vi "extract central core for intensity.vi"() -> ()   [LabVIEW 2020]
uses:
  <vilib>/Math Plots/3D Math Plots/3D Surface/3D Surface XCtrl/3D Surface.xctl
  <vilib>/Math Plots/3D Math Plots/3D Surface/3D Surface Datatype/Public/Plot Helper (Vector).vi
  <vilib>/Math Plots/3D Math Plots/3D Surface/3D Surface Datatype/3D Surface Datatype.lvclass
panel:
  in  "Offset Dim 2":i32
  in  "Offset Dim 1":i32
  out "Main Image 2":T1(plugin-control)
  out "Core Image":T1(plugin-control)
  in  "Boolean":bool
  out "3D Surface":refnum<class "3D Plot Datatype.lvclass">[](xcontrol)
  in  "Intensity Graph colour palette":cluster{dbl, "Color Box":u32}[](array[cluster])=[{1000.0, "Color Box"=16714752}, {750.0, "Color Box"=15859456}, {500.0, "Color Box"=65289}, {250.0, "Color Box"=983260}, {0.0, "Color Box"=14418124}]
  out "output array":i16[](array[numeric])
  out "Intensity Graph 3":i16[][](graph)
  out "dim2_length":i32
  out "dim2_start":i32
  out "dim1_length":i32
  out "dim1_start":i32
  in  "Core extraction size":i32
  out "output variable 6":dbl
  out "output variable 5":dbl
  out "output variable 4":dbl
  out "output variable 3":dbl
  out "output variable 2":i32
  out "output variable":i32
  out "size(s)":i32[](array[numeric])
  out "Intensity Graph 2":i16[][](graph)
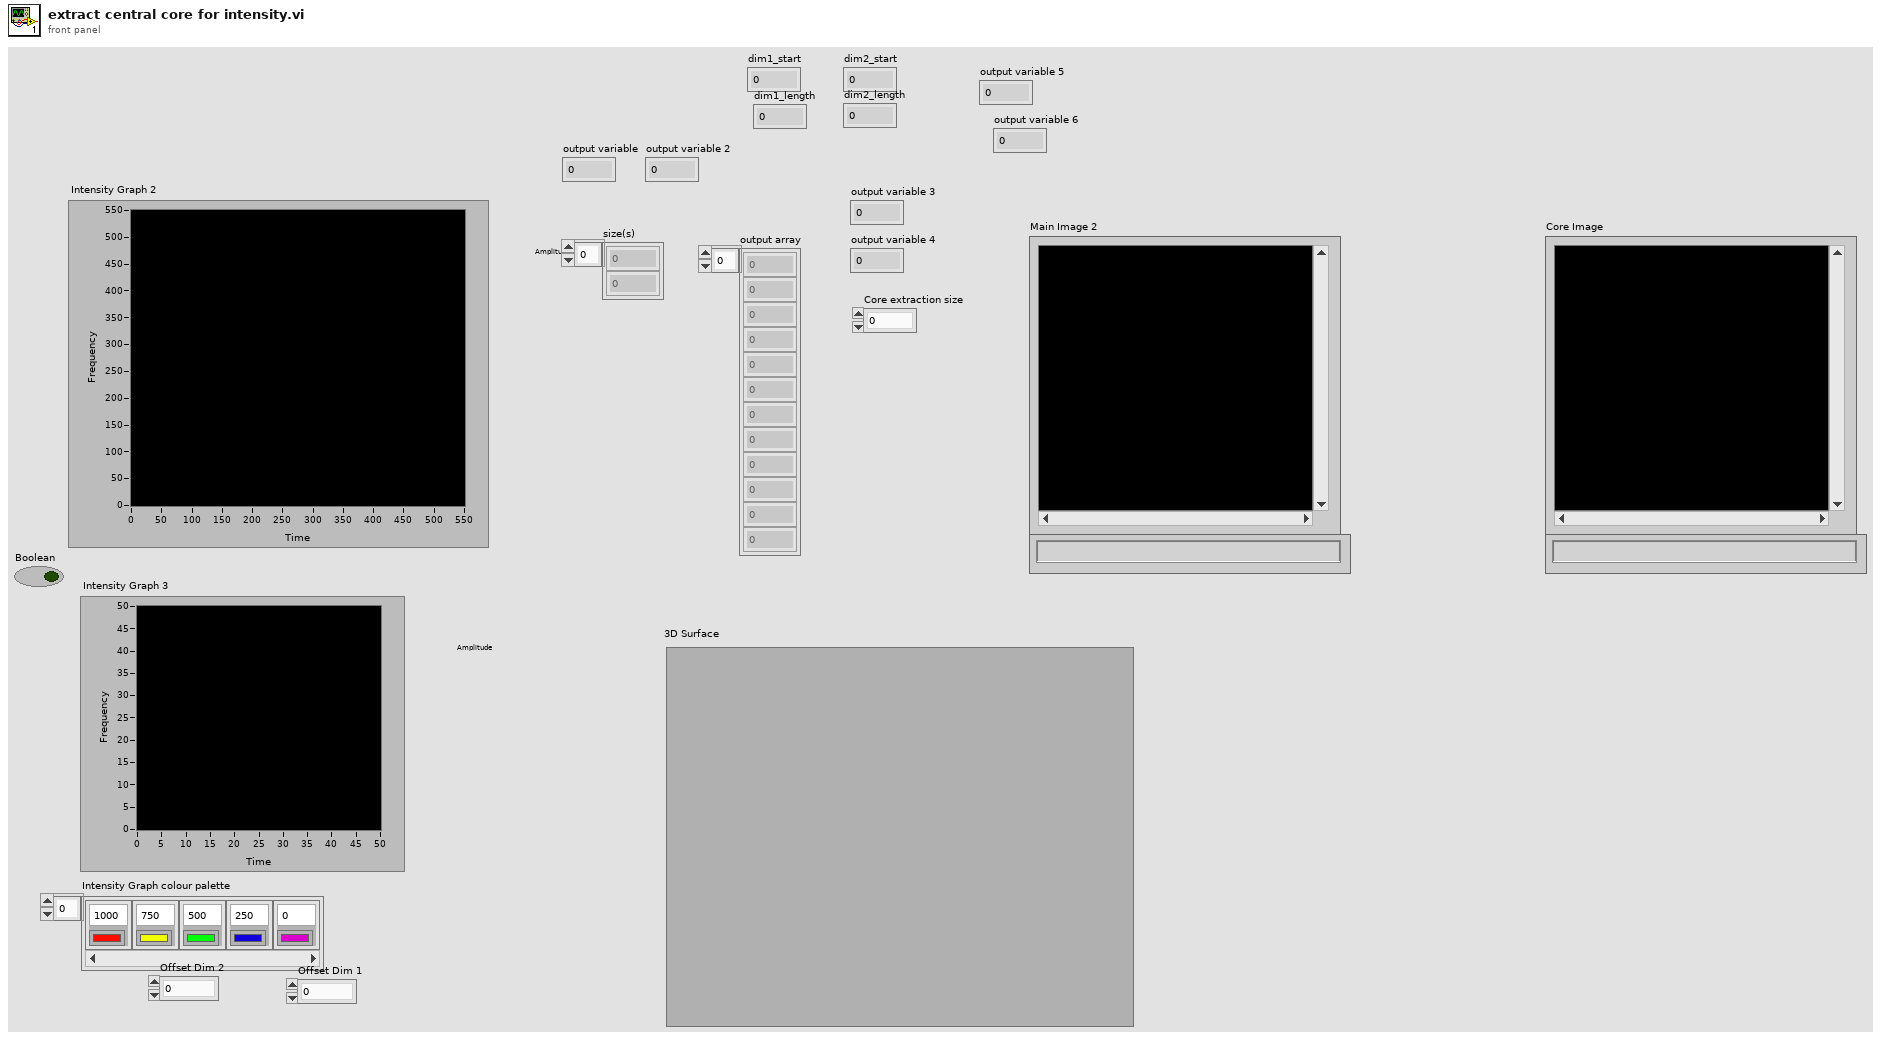
[diagram p1: front panel]
types:
  T1 = typedef "IMAQ Image.ctl" = refnum<image>
  T2 = cluster{"Left":i32, "Top":i32, "Right":i32, "Bottom":i32}
  T3 = typedef "Image Type" = u32
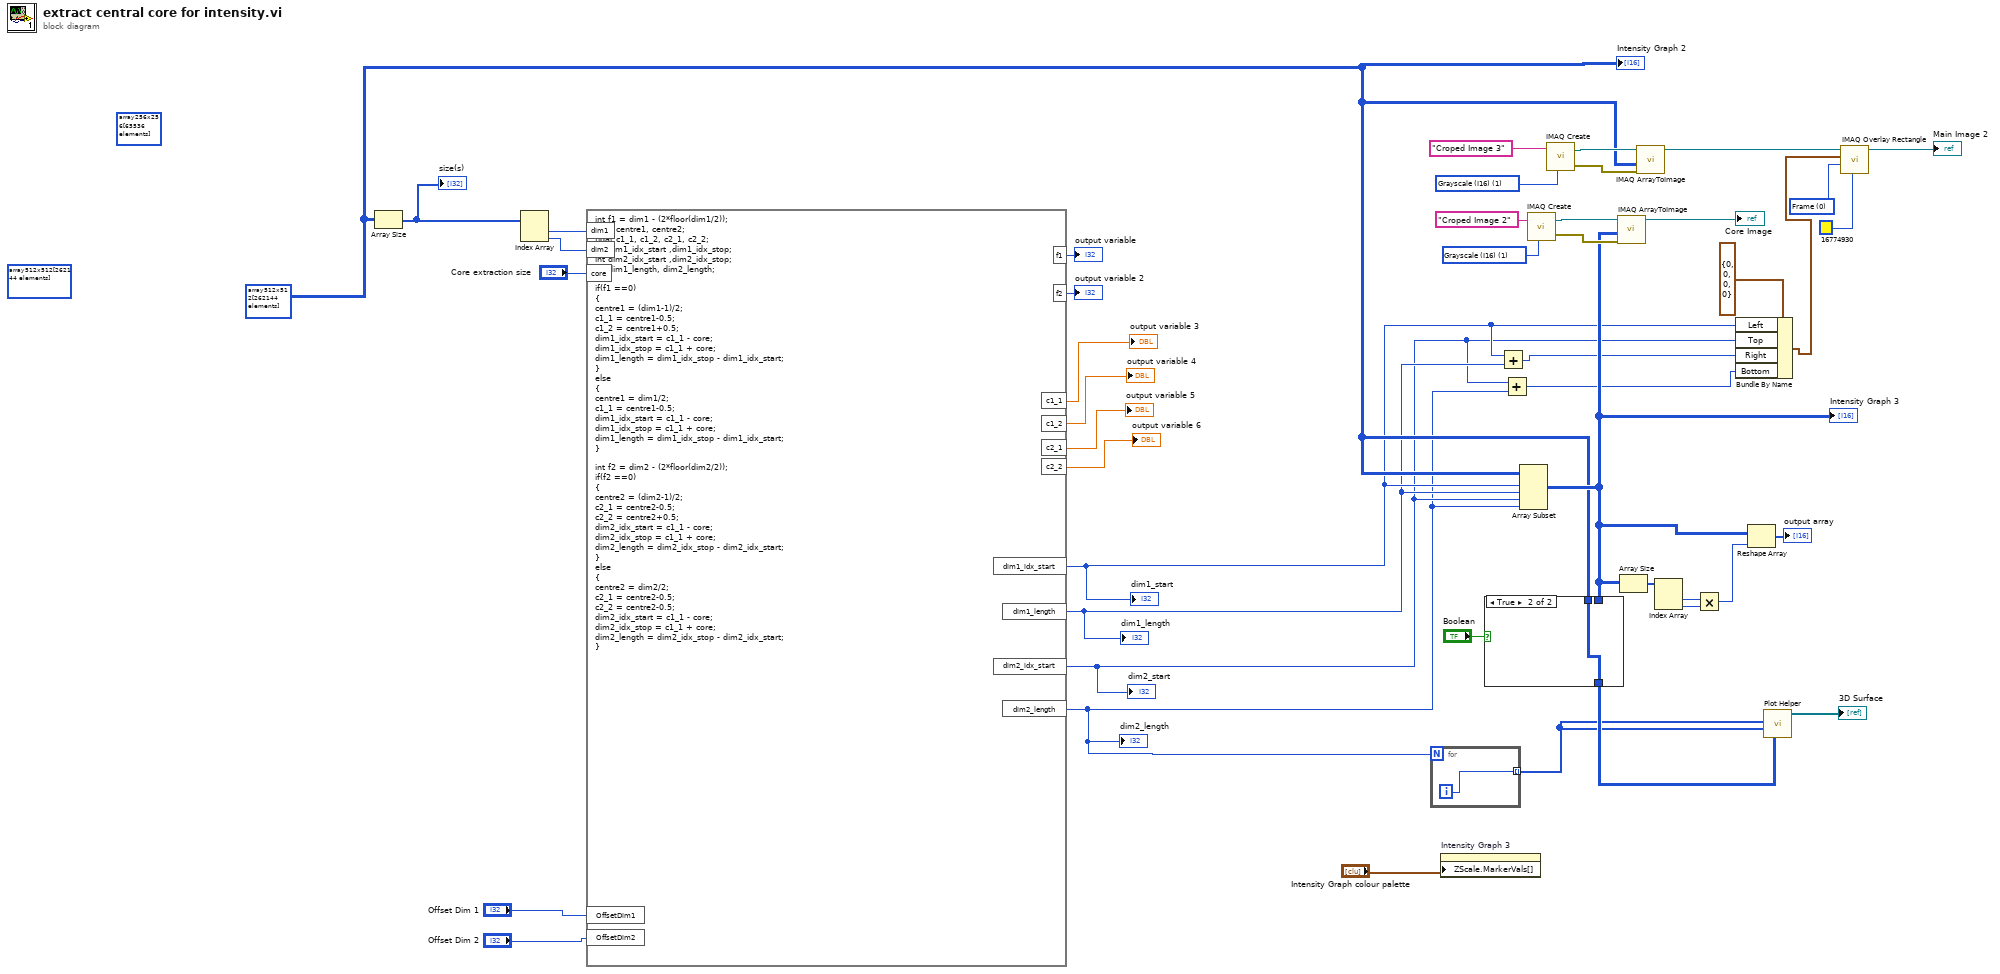
[diagram p0: block diagram]
diagram:
  w12 = u32 0 items=["Frame", "Fill", "Highlight"] ("Drawing Mode (Frame)")
  w17 = T3 1 items=["Grayscale (U8)", "Grayscale (I16)", "Grayscale (SGL)", "Complex (CSG)", "RGB (U32)", "HSL (U32)", "RGB (U64)", "Grayscale (U16)"] ("Image Type")
  w24 = T3 1 items=["Grayscale (U8)", "Grayscale (I16)", "Grayscale (SGL)", "Complex (CSG)", "RGB (U32)", "HSL (U32)", "RGB (U64)", "Grayscale (U16)"] ("Image Type")
  (unwired) i16[][] array256x256[65536 elements] ("Image Pixels (I16)")
  w15 = i16[][] array512x512[262144 elements] ("Image Pixels (I16)")
  (unwired) i16[][] array512x512[262144 elements] ("Intensity Graph 3")
  n1 = Array Size(array=w15) -> (size(s)=w45:i32[])
  "size(s)" <- w45
  n2 = Index Array(array=w45) -> (element #1=w44:i32, element #2=w43:i32)  [unwired: 2 in]
  n3 = formula code="int f1 = dim1 - (2*floor(dim1/2));\nfloat centre1, centre2;\nfloat c1_1, c1_2, c2_1, c2_2;\nint dim1_idx_start ,dim1_idx_stop;\nint dim2_idx_start ,dim2_idx_stop;\nint dim1_length, dim2_length;\n\nif(f1 ==0)\n{\ncentre1 = (dim1-1)/2;\nc1_1 = centre1-0.5;\nc1_2 = centre1+0.5;\ndim1_idx_start = c1_1 - core;\ndim1_idx_stop = c1_1 + core;\ndim1_length = dim1_idx_stop - dim1_idx_start;\n}\nelse\n{\ncentre1 = dim1/2;\nc1_1 = centre1-0.5;\ndim1_idx_start = c1_1 - core;\ndim1_idx_stop = c1_1 + core;\ndim1_length = dim1_idx_stop - dim1_idx_start;\n}\n\nint f2 = dim2 - (2*floor(dim2/2));\nif(f2 ==0)\n{\ncentre2 = (dim2-1)/2;\nc2_1 = centre2-0.5;\nc2_2 = centre2+0.5;\ndim2_idx_start = c1_1 - core;\ndim2_idx_stop = c1_1 + core;\ndim2_length = dim2_idx_stop - dim2_idx_start;\n}\nelse\n{\ncentre2 = dim2/2;\nc2_1 = centre2-0.5; \nc2_2 = centre2-0.5;\ndim2_idx_start = c1_1 - core;\ndim2_idx_stop = c1_1 + core;\ndim2_length = dim2_idx_stop - dim2_idx_start;\n}"("dim1"=w44, "dim2"=w43, "core"="Core extraction size", "OffsetDim1"="Offset Dim 1", "OffsetDim2"="Offset Dim 2") -> ("f1"=→"output variable":i32, "f2"=→"output variable 2":i32, "c1_1"=→"output variable 3":dbl, "c1_2"=→"output variable 4":dbl, "c2_1"=→"output variable 5":dbl, "c2_2"=→"output variable 6":dbl, "dim1_idx_start"=w8:i32, "dim1_length"=w7:i32, "dim2_idx_start"=w5:i32, "dim2_length"=w4:i32)
  "dim1_start" <- w8
  "dim1_length" <- w7
  "dim2_start" <- w5
  "dim2_length" <- w4
  n4 = for {
    N: w4 -> [_]
    tunnel: [w46] -> w26 mode=indexing
    i -> [w46]
  }
  n5 = property on="Intensity Graph 3" class="IntGraph (strict)"("ZScale.MarkerVals[]"="Intensity Graph colour palette") -> ()  [unwired: 2 in, 2 out]
  n6 = Add(x=w8, y=w7) -> (x+y=w6:i32)
  n7 = Add(x=w5, y=w4) -> (x+y=w3:i32)
  n8 = Array Subset(array=w15, index (row)=w8, length (row)=w7, index (col)=w5, length (col)=w4) -> (w20:i16[][])
  "Intensity Graph 3" <- w20
  n9 = case shown="True" "Boolean" {
    tunnel: w20 -> [w47 _]
    tunnel: [w47 w48] -> w28
    tunnel: w15 -> [_ w48]
    frame False {
    }
    frame True {
    }
  }
  n10 = call "IMAQ Create"("Image Name"="Croped Image 2", "Image Type"=w24) -> ("New Image"=w23:T1, "error out"=w22:errorcluster)  [unwired: 3 in]
  n11 = call "IMAQ Create"("Image Name"="Croped Image 3", "Image Type"=w17) -> ("New Image"=w18:T1, "error out"=w19:errorcluster)  [unwired: 3 in]
  n12 = call "IMAQ ArrayToImage"("error in (no error)"=w22, "Image Pixels (I16)"=w20, "Image"=w23) -> ("Image Out"=→"Core Image":T1)  [unwired: 7 in, 1 out]
  n13 = Array Size(array=w20) -> (size(s)=w34:i32[])
  n14 = call "IMAQ ArrayToImage"("error in (no error)"=w19, "Image Pixels (I16)"=w15, "Image"=w18) -> ("Image Out"=w14:T1)  [unwired: 7 in, 1 out]
  n15 = Index Array(array=w34) -> (element #1=w33:i32, element #2=w32:i32)  [unwired: 2 in]
  n16 = Multiply(x=w33, y=w32) -> (x*y=w31:i32)
  n17 = Bundle By Name(cluster=T2 {"Left"=0, "Top"=0, "Right"=0, "Bottom"=0} ("Rectangle"), "Left"=w8, "Top"=w5, "Right"=w6, "Bottom"=w3) -> (w9:T2)
  n18 = Reshape Array(w20, w31) -> (→"output array":i16[])
  n19 = call-poly <vilib>:"Plot Helper.vi"("z matrix"=w28, "y vector"=w26, "x vector"=w26) -> ("3D Plot lvclass Array out"=→"3D Surface":refnum<class "3D Plot Datatype.lvclass">[])  [unwired: 3 in, 5 out]
  n20 = call "IMAQ Overlay Rectangle"("Color"=u32 16774930, "Drawing Mode (Frame)"=w12, "Rectangle"=w9, "Image"=w14) -> ("Image Out"=→"Main Image 2":T1)  [unwired: 6 in, 1 out]
  "Intensity Graph 2" <- w15
